vi "servo.labview.vi"() -> ()   [LabVIEW 2026]
uses:
  <vilib>/Instr/_visa.llb/VISA Configure Serial Port (Instr).vi
panel:
  out "decimal integer string":string
  in  "Gauge":dbl(knob) caption="servo angle" scale=0.1..100.0
  in  "stop":bool
  in  "VISA resource name":refnum<visa-resource-name>
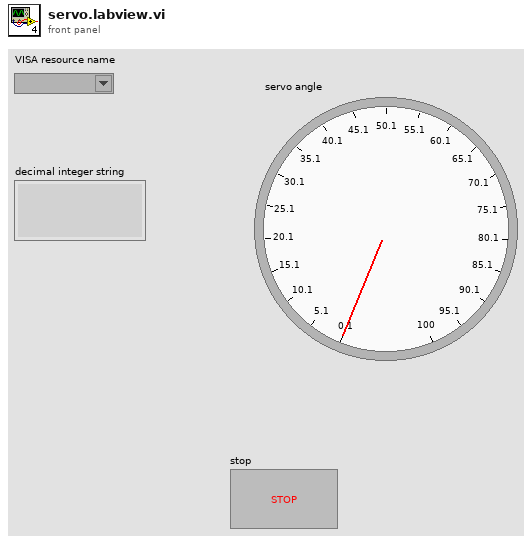
[diagram p1: front panel]
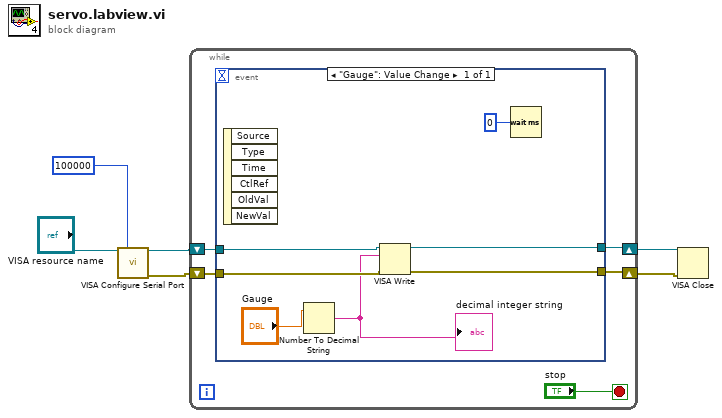
[diagram p0: block diagram]
diagram:
  n1 = call-poly "VISA Configure Serial Port"("VISA resource name"="VISA resource name", "timeout (10sec)"=u32 100000) -> ("VISA resource name out"=w4:refnum<visa-resource-name>, "error out"=w3:errorcluster)  [unwired: 12 in]
  n2 = while {
    shift-right: [w9] -> w2
    shift-left: w4 -> [w11]
    shift-right: [w8] -> w1
    shift-left: w3 -> [w10]
    stop <- "stop" stop-if-true
    n3 = event shown="[0] \"Gauge\": Value Change" {
      selector: _ -> [_]
      dyn-events: _ -> [_]
      timeout: _ -> [_]
      tunnel: w11 -> [w12]
      tunnel: w10 -> [w18]
      tunnel: [w17] -> w9
      tunnel: [w16] -> w8
      event "Gauge": Value Change {
        n4 = event-data() -> ()  [unwired: 1 in, 6 out]
        n5 = Number To Decimal String(number="Gauge") -> (decimal integer string=w14:string)  [unwired: 1 in]
        "decimal integer string" <- w14
        n6 = VISA Write(VISA resource name=w12, write buffer=w14, error in (no error)=w18) -> (VISA resource name out=w17:refnum<visa-resource-name>, error out=w16:errorcluster)  [unwired: 1 out]
        n7 = Wait (ms)(milliseconds to wait=u32 0) -> ()  [unwired: 1 out]
      }
    }
  }
  n8 = VISA Close(VISA resource name=w2, error in (no error)=w1) -> ()  [unwired: 1 out]
